vi "upg4_penplotter.vi"() -> ()   [LabVIEW 2024]
uses:
  <vilib>/Instr/_visa.llb/VISA Configure Serial Port (Instr).vi
panel:
  out "decimal integer string":string
  out "max value":dbl
  in  "Samplingsintervall":dbl
  in  "Mätvärden":dbl[](array[numeric])
  out "Y-axel":string
  out "X-axel":string
  out "datapunkter":string
  out "error out":errorcluster
  in  "flow control":u16(ring)=4 items=["None"=0, "XON/XOFF"=1, "RTS/CTS"=2, "DTR/DSR"=4]
  in  "stop bits":u16(ring)=10 items=["1.0"=10, "1.5"=15, "2.0"=20]
  in  "parity":u16(ring) items=["None", "Odd", "Even", "Mark", "Space"]
  in  "data bits":u16=8 min=5 max=8 step=1
  in  "VISA resource name":refnum<visa-resource-name>="COM1"
  in  "baud rate":u32=9600
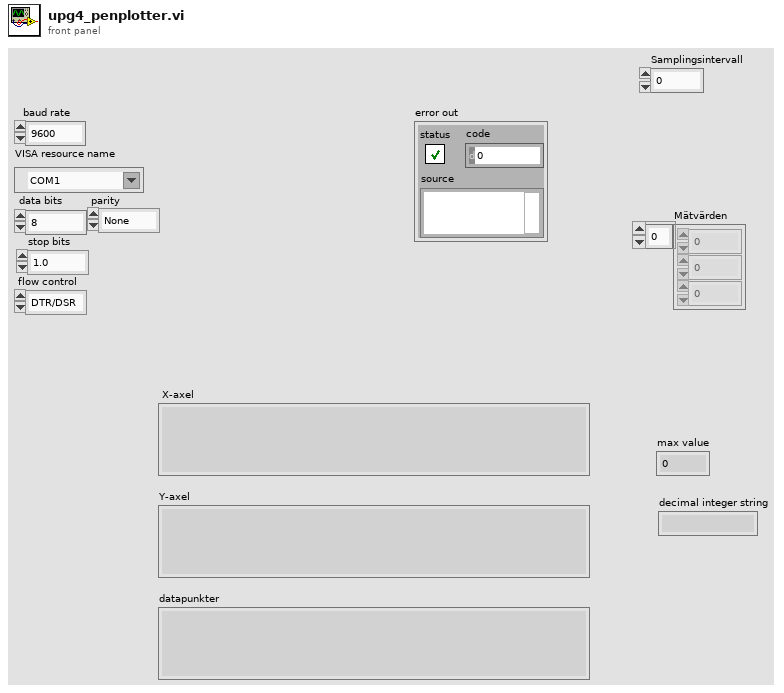
[diagram p1: front panel]
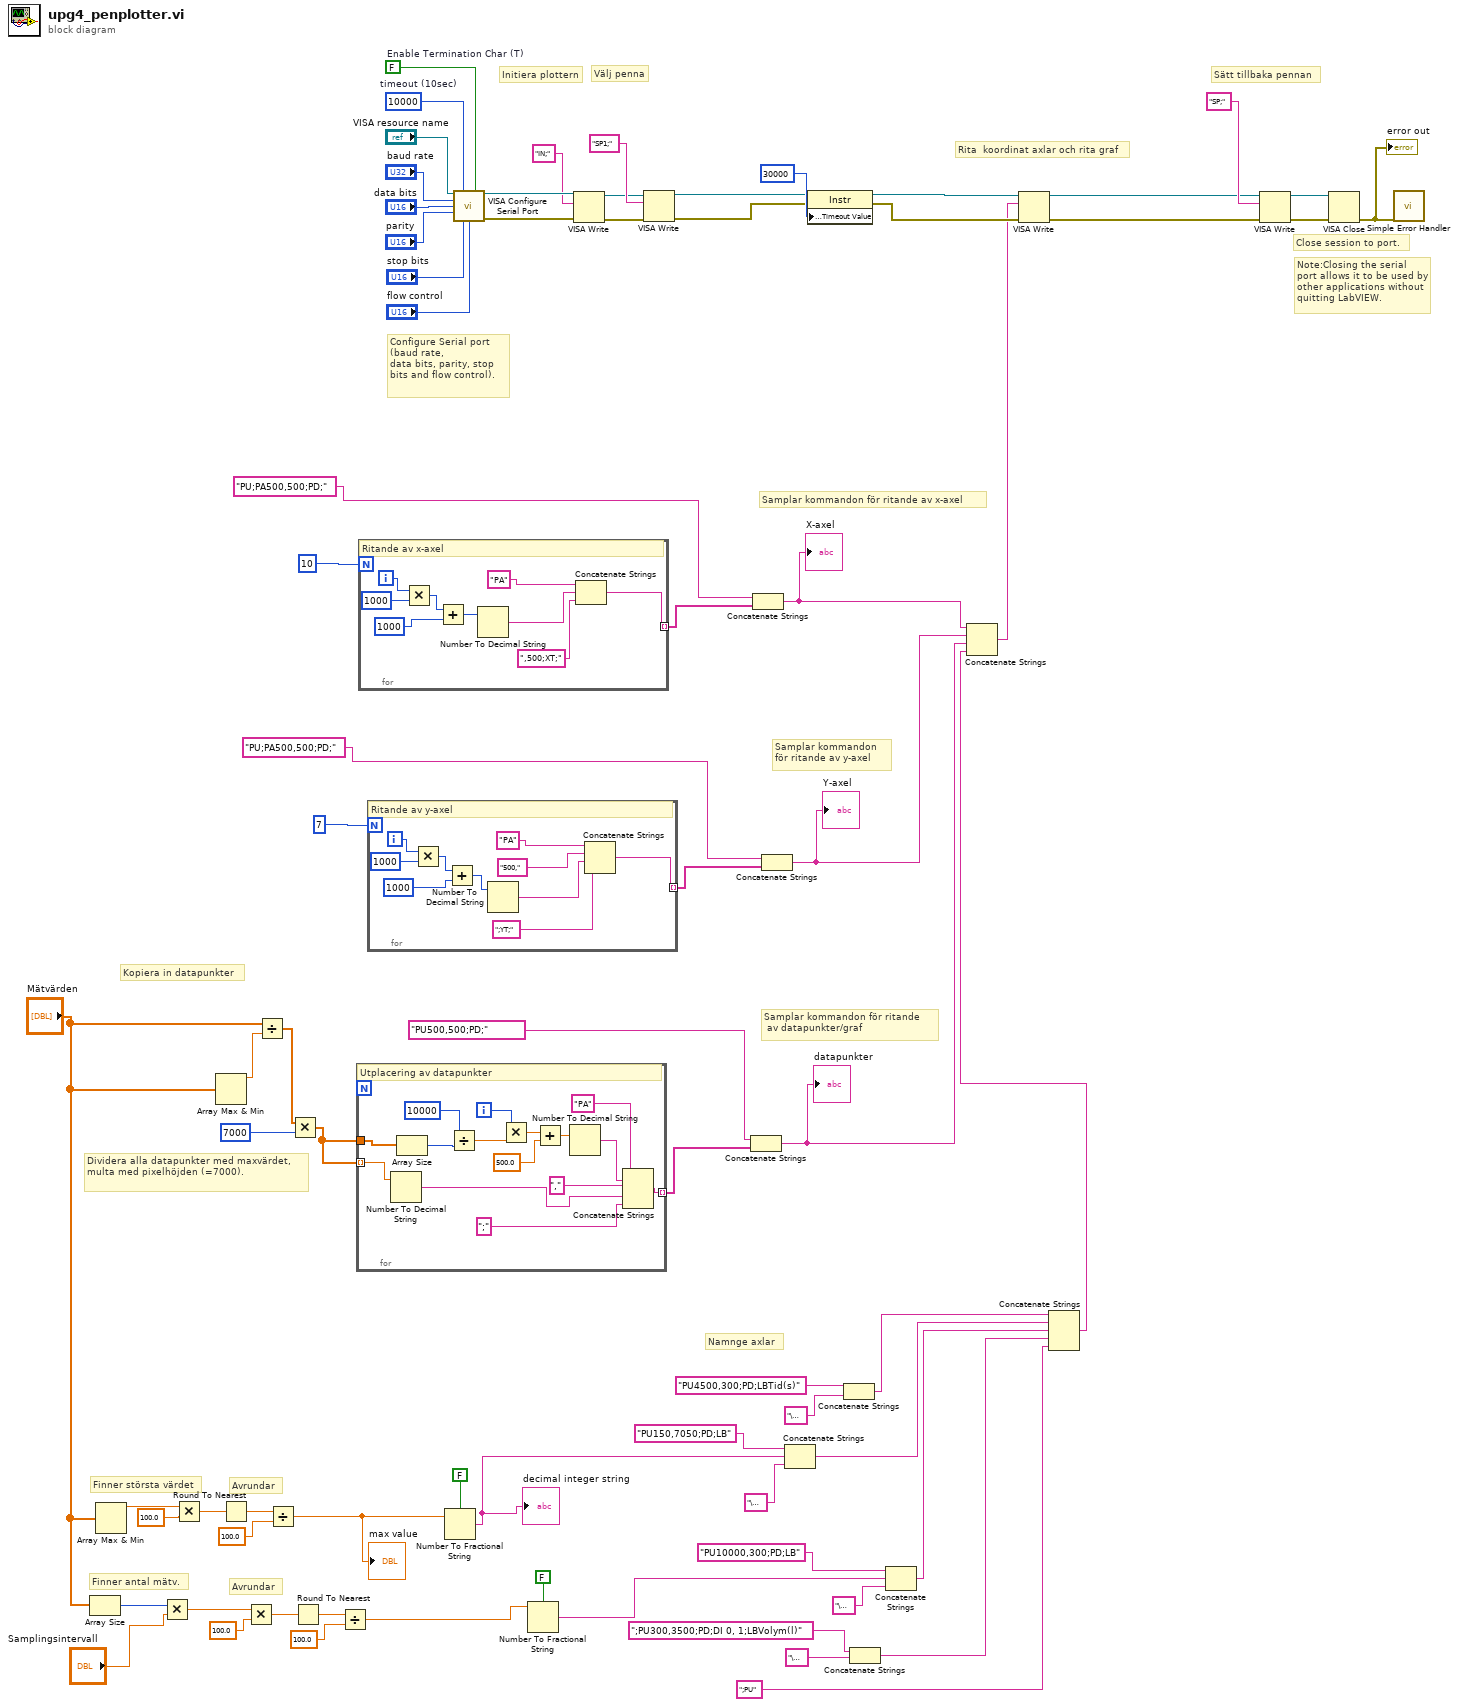
[diagram p0: block diagram]
diagram:
  w69 = FALSE  # Enable Termination Char (T)
  w70 = u32 10000  # timeout (10sec)
  # "Finner antal mätv."
  # "Finner största värdet"
  # "Avrundar"
  # "Avrundar"
  # "Samplar kommandon för ritande\n av datapunkter/graf"
  # "Samplar kommandon\nför ritande av y-axel"
  # "Samplar kommandon för ritande av x-axel"
  # "Namnge axlar"
  # "Dividera alla datapunkter med maxvärdet,\nmulta med pixelhöjden (=7000)."
  # "Kopiera in datapunkter"
  # "Initiera plottern"
  # "Välj penna"
  # "Sätt tillbaka pennan"
  # "Rita  koordinat axlar och rita graf"
  # "Note:Closing the serial port allows it to be used by other applications without\nquitting LabVIEW."
  # "Configure Serial port (baud rate,\ndata bits, parity, stop bits and flow control)."
  # "Close session to port."
  n1 = Array Size(array="Mätvärden") -> (size(s)=w23:i32)
  n2 = Array Max & Min(array="Mätvärden") -> (max value=w12:dbl)  [unwired: 3 out]
  n3 = Multiply(x=w23, y="Samplingsintervall") -> (x*y=w2:dbl)
  n4 = Multiply(x=w12, y=100.0) -> (x*y=w10:dbl)
  n5 = Array Max & Min(array="Mätvärden") -> (max value=w39:dbl)  [unwired: 3 out]
  n6 = Round To Nearest(number=w10) -> (nearest integer value=w9:dbl)
  n7 = Multiply(x=w2, y=100.0) -> (x*y=w5:dbl)
  n8 = Divide(x="Mätvärden", y=w39) -> (x/y=w38:dbl[])
  n9 = Divide(x=w9, y=100.0) -> (x/y=w7:dbl)
  "max value" <- w7
  n10 = Multiply(x=w38, y=7000) -> (x*y=w36:dbl[])
  n11 = Round To Nearest(number=w5) -> (nearest integer value=w4:dbl)
  n12 = Divide(x=w4, y=100.0) -> (x/y=w1:dbl)
  n13 = for {
    tunnel: w36 -> [w89] mode=indexing
    tunnel: w36 -> [w78]
    tunnel: [w81] -> w50 mode=indexing
    i -> [w79]
    # "Utplacering av datapunkter"
    n14 = Number To Decimal String(number=w89) -> (decimal integer string=w84:string)  [unwired: 1 in]
    n15 = Array Size(array=w78) -> (size(s)=w87:i32)
    n16 = Divide(x=10000, y=w87) -> (x/y=w86:dbl)
    n17 = Multiply(x=w79, y=w86) -> (x*y=w76:dbl)
    n18 = Add(x=w76, y=500.0) -> (x+y=w77:dbl)
    n19 = Number To Decimal String(number=w77) -> (decimal integer string=w85:string)  [unwired: 1 in]
    n20 = Concatenate Strings("PA", w85, ",", w84, ";") -> (w81:string)
  }
  n21 = for {
    N: 10 -> [_]
    tunnel: [w90] -> w46 mode=indexing
    i -> [w98]
    # "Ritande av x-axel"
    n22 = Multiply(x=w98, y=1000) -> (x*y=w96:i32)
    n23 = Add(x=w96, y=1000) -> (x+y=w94:i32)
    n24 = Number To Decimal String(number=w94) -> (decimal integer string=w93:string)  [unwired: 1 in]
    n25 = Concatenate Strings("PA", w93, ",500;XT;") -> (w90:string)
  }
  n26 = for {
    N: 7 -> [_]
    tunnel: [w102] -> w49 mode=indexing
    i -> [w108]
    # "Ritande av y-axel"
    n27 = Multiply(x=w108, y=1000) -> (x*y=w106:i32)
    n28 = Add(x=w106, y=1000) -> (x+y=w104:i32)
    n29 = Number To Decimal String(number=w104) -> (decimal integer string=w100:string)  [unwired: 1 in]
    n30 = Concatenate Strings("PA", "500,", w100, ";YT;") -> (w102:string)
  }
  n31 = Number To Fractional String(use system decimal point (T)=FALSE, number=w7) -> (F-format string=w14:string)  [unwired: 2 in]
  "decimal integer string" <- w14
  n32 = call-poly "VISA Configure Serial Port"("VISA resource name"="VISA resource name", "timeout (10sec)"=w70, "Enable Termination\nChar (T)"=w69, "baud rate (9600)"="baud rate", "data bits (8)"="data bits", "parity (0:none)"="parity", "stop bits (10: 1 bit)"="stop bits", "flow control (0:none)"="flow control") -> ("VISA resource name out"=w61:refnum<visa-resource-name>, "error out"=w59:errorcluster)  [unwired: 6 in]
  n33 = Number To Fractional String(use system decimal point (T)=FALSE, number=w1) -> (F-format string=w13:string)  [unwired: 2 in]
  n34 = VISA Write(VISA resource name=w61, write buffer="IN;", error in (no error)=w59) -> (VISA resource name out=w60:refnum<visa-resource-name>, error out=w58:errorcluster)  [unwired: 1 out]
  n35 = VISA Write(VISA resource name=w60, write buffer="SP1;", error in (no error)=w58) -> (VISA resource name out=w55:refnum<visa-resource-name>, error out=w54:errorcluster)  [unwired: 1 out]
  n36 = Concatenate Strings("PU500,500;PD;", w50) -> (w41:string)
  "datapunkter" <- w41
  n37 = Concatenate Strings("PU;PA500,500;PD;", w46) -> (w43:string)
  "X-axel" <- w43
  n38 = Concatenate Strings("PU;PA500,500;PD;", w49) -> (w42:string)
  "Y-axel" <- w42
  n39 = Concatenate Strings("PU150,7050;PD;LB" ("string"), w14, "\u0003") -> (w20:string)
  n40 = property class="Instr"(reference=w55, error in=w54, "General Settings:Timeout Value"=u32 30000) -> (reference out=w53:refnum<visa-resource-name>, error out=w52:errorcluster)
  n41 = Concatenate Strings("PU4500,300;PD;LBTid(s)" ("string"), "\u0003") -> (w21:string)
  n42 = Concatenate Strings(";PU300,3500;PD;DI 0, 1;LBVolym(l)" ("string"), "\u0003") -> (w18:string)
  n43 = Concatenate Strings("PU10000,300;PD;LB" ("string"), w13, "\u0003") -> (w19:string)
  n44 = Concatenate Strings(w21, w20, w19, w18, ";PU") -> (w29:string)
  n45 = Concatenate Strings(w43, w42, w41, w29) -> (w40:string)
  n46 = VISA Write(VISA resource name=w53, write buffer=w40, error in (no error)=w52) -> (VISA resource name out=w35:refnum<visa-resource-name>, error out=w34:errorcluster)  [unwired: 1 out]
  n47 = VISA Write(VISA resource name=w35, write buffer="SP;", error in (no error)=w34) -> (VISA resource name out=w64:refnum<visa-resource-name>, error out=w65:errorcluster)  [unwired: 1 out]
  n48 = VISA Close(VISA resource name=w64, error in (no error)=w65) -> (error out=w72:errorcluster)
  "error out" <- w72
  n49 = call <vilib>:"Simple Error Handler.vi"("error in (no error)"=w72) -> ()  [unwired: 4 in, 5 out]
